vi "Reset.vi"(8 "error in (no error)":errorcluster, 11 "ID in":refnum<class "ID.lvclass">) -> (0 "error out":errorcluster, 3 "ID out":refnum<class "ID.lvclass">)   [LabVIEW 2020, in "ID.lvclass"]
uses:
  ID.lvclass
  Controller/Ctrl_ID.ctl
  ID.lvclass/ID.ctl
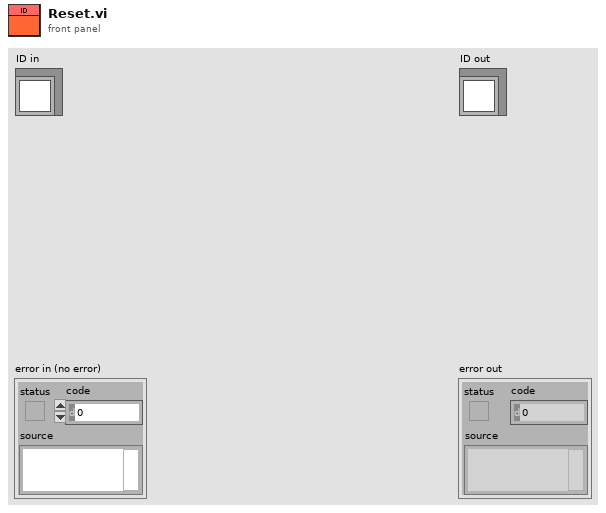
[diagram p1: front panel]
types:
  T1 = typedef "Ctrl_ID.ctl" = cluster{"Nom":string, "Prenom":string, "Age":u8, "Sex":bool}
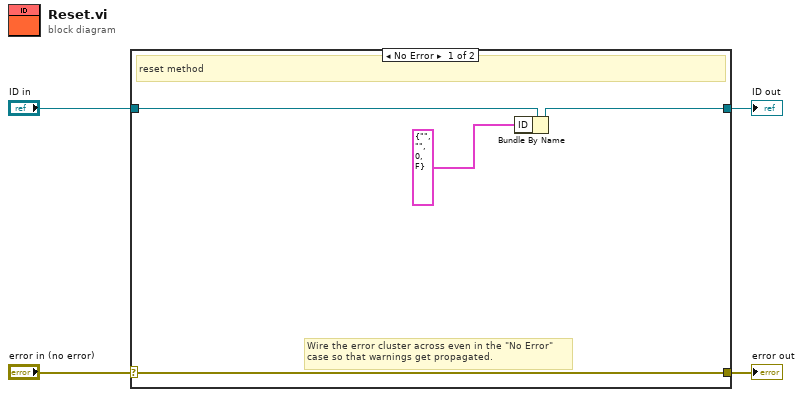
[diagram p0: block diagram]
diagram:
  n1 = case shown="No Error" "error in (no error)" {
    selector: "error in (no error)" -> [w7 w10]
    tunnel: [w7 w10] -> w3
    tunnel: [w6 w9] -> w1
    tunnel: "ID in" -> [w8 w9]
    frame No Error {
      # "Wire the error cluster across even in the \"No Error\"\ncase so that warnings get propagated."
      # "reset method"
      n2 = Bundle By Name(cluster=w8, "ID"=T1 {"Nom"="", "Prenom"="", "Age"=0, "Sex"=FALSE}) -> (w6:refnum<class "ID.lvclass">)
    }
    frame Error {
    }
  }
  "error out" <- w3
  "ID out" <- w1
